vi "watch(real time).vi"() -> ()   [LabVIEW 2009]
uses:
  <vilib>/Utility/file.llb/Read From Spreadsheet File (DBL).vi
  <vilib>/vision/NI_Vision_Development_Module.lvlib
panel:
  in  "stop":bool
  in  "Play":bool
  in  "before":u8(slide)=2 scale=20.0..0.0
  in  "after":u8(slide)=2 scale=0.0..20.0
  in  "EDIT VIDEO":bool
  in  "BADS":bool
  out "DISP":T1(plugin-control)
  out "TIME intervals":dbl[](array[numeric])
  in  "Vid file":path caption="Open AVI file"
  out "TIME selected events":dbl[](array[numeric])
  out "DATA selected events":dbl[][](array[numeric])
  out "coded data":dbl[][](array[numeric])
  out "time data":dbl[](array[numeric])
  out "DATA IN":dbl[][](array[numeric]) format="%0.3f"
  in  "Data file":path caption="Read data from"
  out "EVENTS":bool[](array[boolean])
  in  "PivF":bool
  in  "ShArm":bool
  in  "REB":bool
  in  "OFF":bool
  in  "DEF":bool
  in  "3PT":bool
  in  "2PT":bool
  in  "SHOT":bool
  in  "BLK":bool
  in  "TUR":bool
  in  "AST":bool
  in  "SF":bool
  in  "C":bool
  in  "PF":bool
  in  "PG":bool
  in  "SG":bool
  # "PLAYER"
  # "Playback interval (s)"
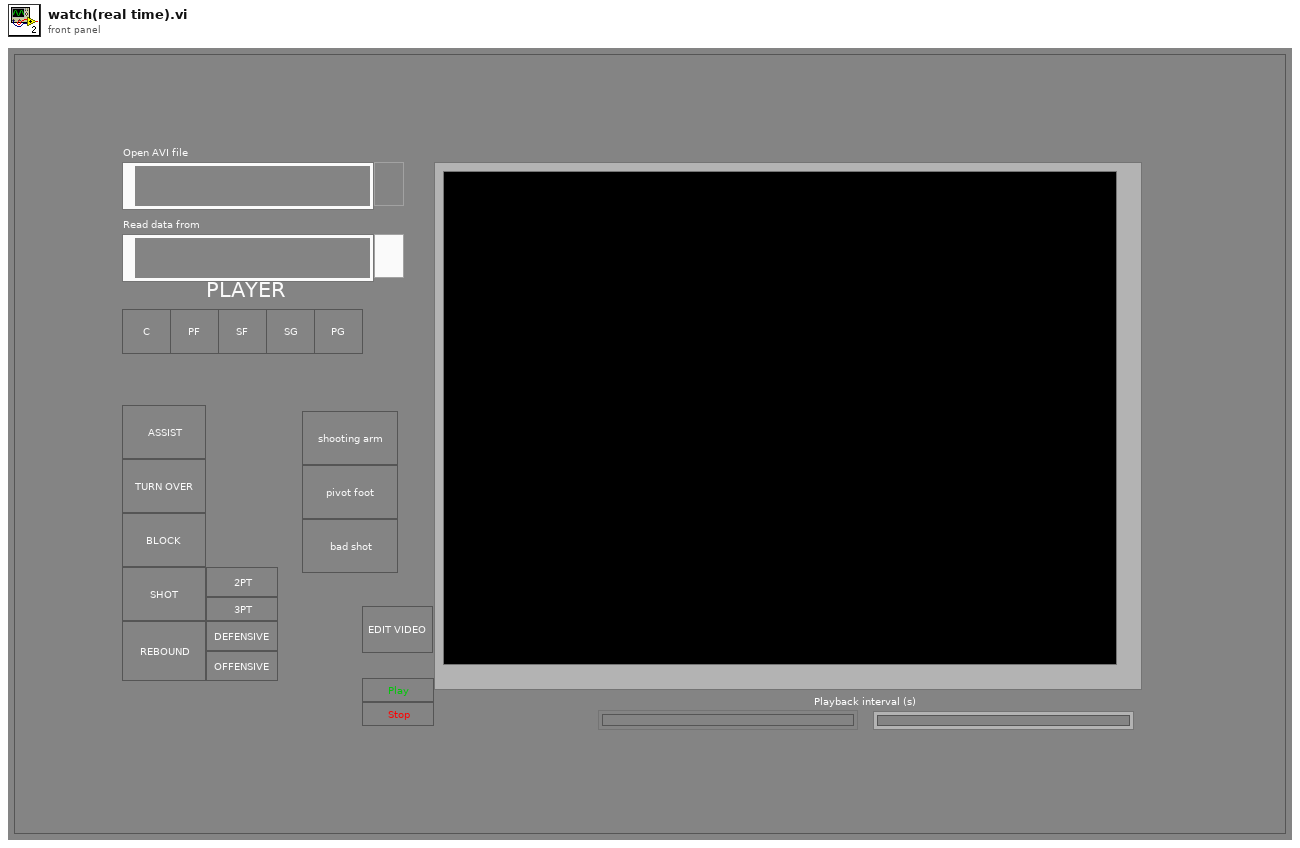
[diagram p1: front panel]
types:
  T1 = typedef "IMAQ Image.ctl" = refnum<image>
  T2 = typedef "Image Type" = u32
  T3 = typedef "AviRefnum.ctl" = refnum<k1>
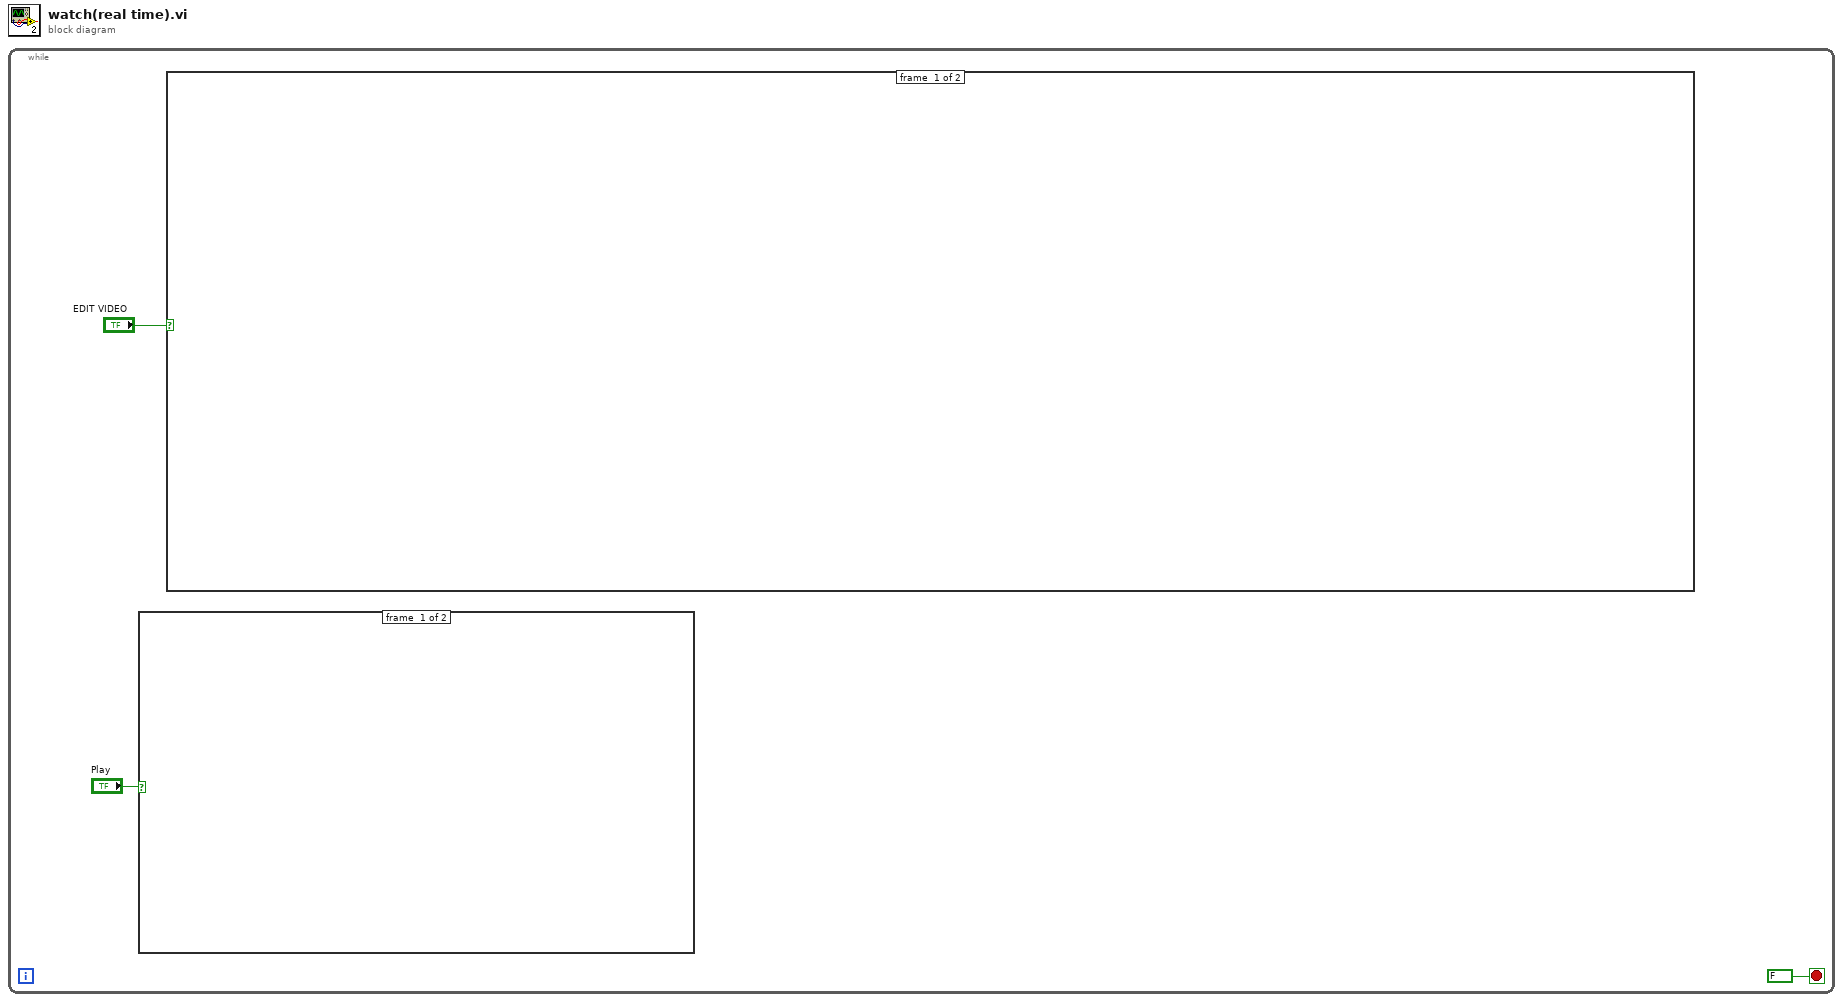
[diagram p0: block diagram]
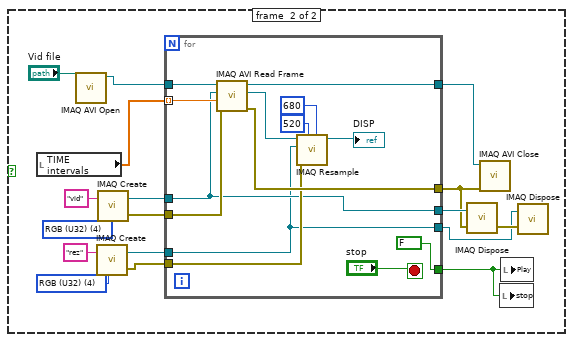
[diagram p2: hidden frame]
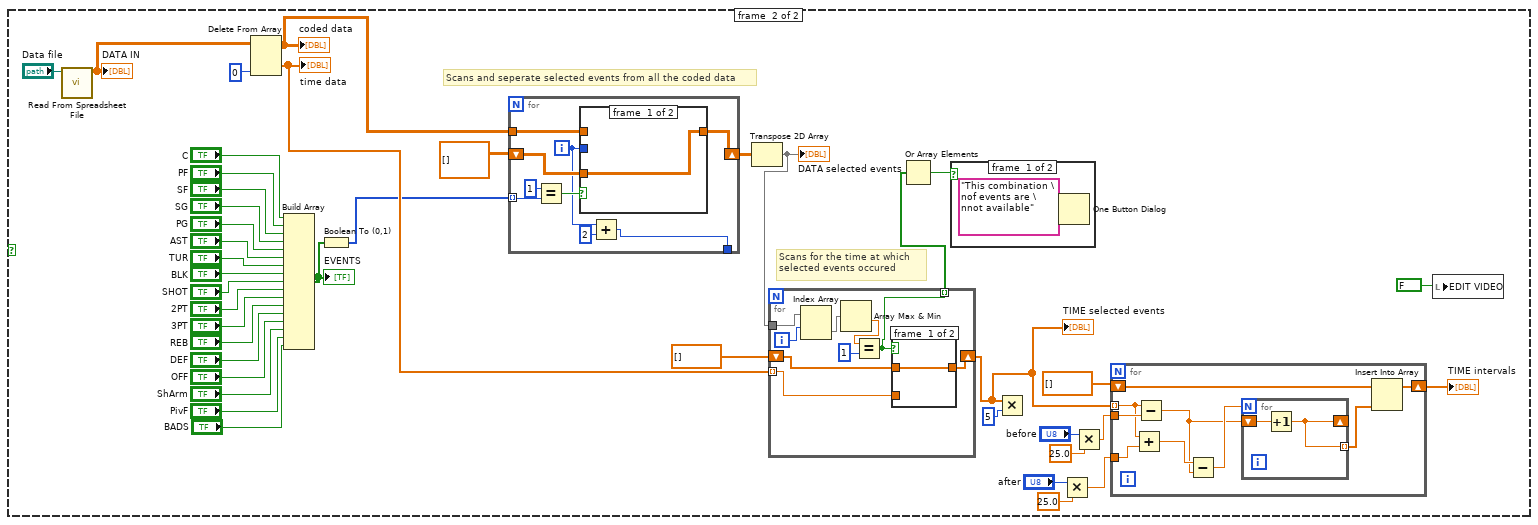
[diagram p3: hidden frame]
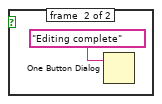
[diagram p4: hidden frame]
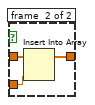
[diagram p5: hidden frame]
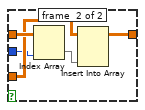
[diagram p6: hidden frame]
diagram:
  n1 = while {
    stop <- FALSE stop-if-true
    n2 = case shown="True" "Play" {
      frame #0 {
      }
      frame #1 {
        w8 = T2 4 items=["Grayscale (U8)", "Grayscale (I16)", "Grayscale (SGL)", "Complex (CSG)", "RGB (U32)", "HSL (U32)", "RGB (U64)", "Grayscale (U16)"] ("Image Type")
        w9 = T2 4 items=["Grayscale (U8)", "Grayscale (I16)", "Grayscale (SGL)", "Complex (CSG)", "RGB (U32)", "HSL (U32)", "RGB (U64)", "Grayscale (U16)"] ("Image Type")
        n3 = local read "TIME intervals"() -> (w18:dbl[])
        n4 = call "IMAQ AVI Open"("AVI Path"="Vid file") -> ("Avi Refnum"=w19:T3)  [unwired: 9 in, 1 out]
        n5 = call "IMAQ Create"("Image Name"="rez", "Image Type"=w8) -> ("New Image"=w12:T1, "error out"=w11:errorcluster)  [unwired: 3 in]
        n6 = call "IMAQ Create"("Image Name"="vid", "Image Type"=w9) -> ("New Image"=w17:T1, "error out"=w15:errorcluster)  [unwired: 3 in]
        n7 = for {
          tunnel: w19 -> [w34]
          tunnel: w18 -> [w33] mode=indexing
          tunnel: w17 -> [w22]
          tunnel: w15 -> [w32]
          tunnel: [w31] -> w14
          tunnel: [w30] -> w6
          tunnel: w12 -> [w21]
          tunnel: w11 -> [w27]
          tunnel: [FALSE ("Play")] -> w10
          tunnel: [w22] -> w7
          tunnel: [w21] -> w4
          stop <- "stop" stop-if-true
          n8 = call "IMAQ AVI Read Frame"("error in (no error)"=w32, "Frame Number"=w33, "Image"=w22, "Avi Refnum"=w34) -> ("error out"=w30:errorcluster, "Image Out"=w24:T1, "Avi Refnum (duplicate)"=w31:T3)  [unwired: 4 in, 1 out]
          n9 = call "IMAQ Resample"("X Resolution"=680, "Y Resolution"=520, "error in (no error)"=w27, "Image Dst"=w21, "Image Src"=w24) -> ("Image Dst Out"=→"DISP":T1)  [unwired: 5 in, 1 out]
        }
        n10 = call "IMAQ Dispose"("Image"=w7, "error in (no error)"=w6) -> ("error out"=w5:errorcluster)  [unwired: 4 in]
        n11 = call "IMAQ AVI Close"("error in (no error)"=w6, "Avi Refnum"=w14) -> ()  [unwired: 9 in, 1 out]
        n12 = local write "stop"(w10) -> ()
        n13 = local write "Play"(w10) -> ()
        n14 = call "IMAQ Dispose"("Image"=w4, "error in (no error)"=w5) -> ()  [unwired: 4 in, 1 out]
      }
    }
    n15 = case shown="True" "EDIT VIDEO" {
      frame #0 {
      }
      frame #1 {
        # "Scans for the time at which \nselected events occured"
        # "Scans and seperate selected events from all the coded data"
        n16 = call-poly <vilib>:"Read From Spreadsheet File.vi"("file path (dialog if empty)"="Data file") -> ("all rows"=w38:dbl[][])  [unwired: 6 in, 4 out]
        "DATA IN" <- w38
        n17 = Delete From Array(array=w38, index (col)=0 ("disabled index (col)")) -> (deleted portion=w60:dbl[], array with subset deleted=w58:dbl[][])  [unwired: 2 in]
        "time data" <- w60
        "coded data" <- w58
        n18 = Build Array("C", "PF", "SF", "SG", "PG", "AST", "TUR", "BLK", "SHOT", "2PT", "3PT", "REB", "DEF", "OFF", "ShArm", "PivF", "BADS") -> (w55:bool[])
        "EVENTS" <- w55
        n19 = Boolean To (0,1)(Boolean=w55) -> (0, 1=w56:i16[])
        n20 = for {
          tunnel: w56 -> [w110] mode=indexing
          shift-right: [w107] -> w59
          shift-left: dbl[][] [] ("array w/ subset deleted") -> [w106]
          tunnel: [w103] -> _
          tunnel: w58 -> [w102]
          i -> [w105]
          n21 = Equal?(x=i16 1, y=w110) -> (x = y?=w108:bool)
          n22 = case shown="True" w108 {
            tunnel: w105 -> [_ w112]
            tunnel: [w111 w114] -> w107
            tunnel: w106 -> [w111 w113]
            tunnel: w102 -> [_ w115]
            frame #0 {
            }
            frame #1 {
              n23 = Index Array(array=w115, index (col)=w112) -> (element=w116:dbl[])  [unwired: 1 in]
              n24 = Insert Into Array(array=w113, new element=w116) -> (w114:dbl[][])  [unwired: 2 in]
            }
          }
          n25 = Add(x=w105, y=2) -> (x+y=w103:i32)
        }
        n26 = Transpose 2D Array(2D array=w59) -> (transposed array=w62:dbl[][])
        "DATA selected events" <- w62
        n27 = for {
          tunnel: w60 -> [w95] mode=indexing
          shift-right: [w94] -> w35
          shift-left: dbl[] [] ("array w/ subset deleted") -> [w96]
          tunnel: w62 -> [w93]
          tunnel: [w89] -> w65 mode=indexing
          i -> [w90]
          n28 = Index Array(array=w93, index (row)=w90) -> (element=w92:dbl[])  [unwired: 1 in]
          n29 = Array Max & Min(array=w92) -> (min value=w91:dbl)  [unwired: 3 out]
          n30 = Equal?(x=w91, y=1) -> (x = y?=w89:bool)
          n31 = case shown="True" w89 {
            tunnel: w96 -> [w98 w101]
            tunnel: w95 -> [_ w100]
            tunnel: [w98 w99] -> w94
            frame #0 {
            }
            frame #1 {
              n32 = Insert Into Array(array=w101, new element=w100) -> (w99:dbl[])  [unwired: 1 in]
            }
          }
        }
        "TIME selected events" <- w35
        n33 = Or Array Elements(Boolean array=w65) -> (logical OR=w64:bool)
        n34 = case shown="True" w64 {
          frame #0 {
            n35 = One Button Dialog(message="This combination \nof events are \nnot available") -> ()  [unwired: 1 in, 1 out]
          }
          frame #1 {
            n36 = One Button Dialog(message="Editing complete") -> ()  [unwired: 1 in, 1 out]
          }
        }
        n37 = Multiply(x=w35, y=5) -> ()  [unwired: 1 out]
        n38 = Multiply(x="after", y=25.0) -> (x*y=w72:dbl)
        n39 = Multiply(x="before", y=25.0) -> (x*y=w71:dbl)
        n40 = for {
          tunnel: w35 -> [w82] mode=indexing
          tunnel: w71 -> [w84]
          tunnel: w72 -> [w83]
          shift-right: [w80] -> w74
          shift-left: dbl[] [] -> [w81]
          n41 = Add(x=w82, y=w83) -> (x+y=w79:dbl)
          n42 = Subtract(x=w82, y=w84) -> (x-y=w77:dbl)
          n43 = Subtract(x=w79, y=w77) -> (x-y=w78:dbl)
          n44 = for {
            N: w78 -> [_]
            shift-right: [w85] -> _
            shift-left: w77 -> [w86]
            tunnel: [w85] -> w76 mode=indexing
            n45 = Increment(x=w86) -> (x+1=w85:dbl)
          }
          n46 = Insert Into Array(array=w81, new element=w76) -> (w80:dbl[])  [unwired: 1 in]
        }
        "TIME intervals" <- w74
        n47 = local write "EDIT VIDEO"(FALSE ("EDIT VIDEO")) -> ()
      }
    }
  }
